vi "Reanimate.vi"(4 "Hook Search Path":path[](array[path]), 6 "Execute Hooks?":cluster{"Pre":bool, "Post":bool}={"Pre"=TRUE, "Post"=TRUE}, 8 "Error In":errorcluster, 10 "Graves":refnum<vi>[](array[refnum]), 11 "VI In":refnum<vi>) -> (0 "Error Out":errorcluster, 2 "Change Made?":bool, 3 "VI Out":refnum<vi>)   [LabVIEW 2018, in "Toolkit.lvlib"]
doc: "Creates zombies at each grave. Enables the Corpse (legacy) frame and disables the Spirit (refactored) frame of each grave. A grave is Diagram Disable Structure with a RIP bookmark tag for its label, a.k.a. tombstone. The Corpse (legacy) frame's subdiagram label is changed from \"Corpse\" to a Zombie bookmark tag with an ISO-8601 timestamp for its \"rebirthday\" and the user that created the zombie, a.k.a. the necromancer, surrounded by parentheses."
uses:
  Toolkit.lvlib
  Typedefs/Bookmark Tags.ctl
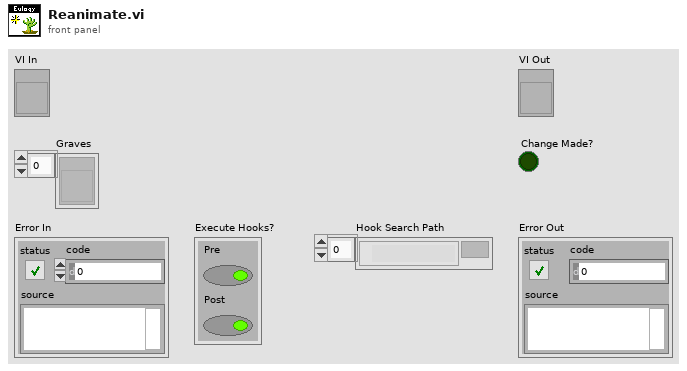
[diagram p1: front panel]
types:
  T1 = typedef "Toolkit.lvlib/Bookmark Tags.ctl" = enum16{"RIP", "Zombie"}
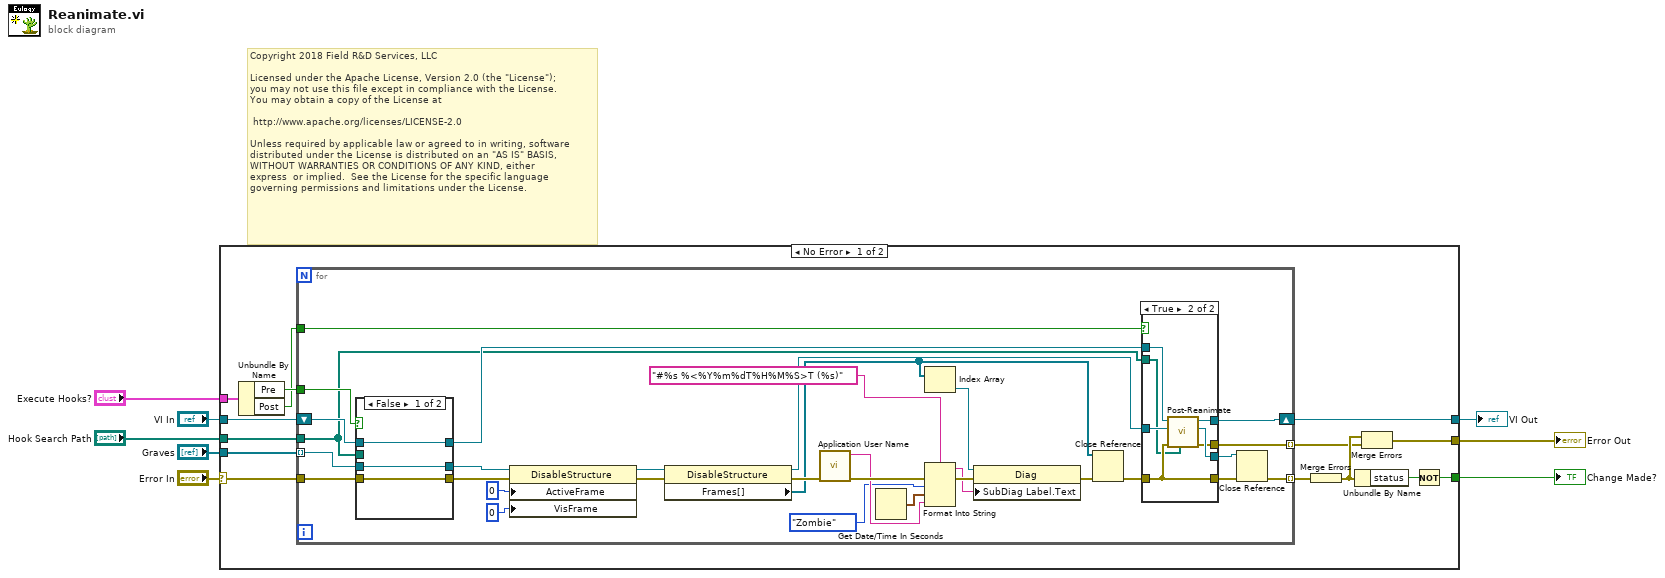
[diagram p0: block diagram]
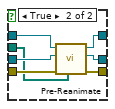
[diagram p3: hidden frame]
diagram:
  # "Copyright 2018 Field R&D Services, LLC\n\nLicensed under the Apache License, Version 2.0 (the \"License\");\nyou may not use this file except in compliance with the License.\nYou may obtain a copy of the License at\n\n\thttp://www.apache.org/licenses/LICENSE-2.0\n\nUnless required by applicable law or agreed to in writing, software\ndistributed under the License is distributed on an \"AS IS\" BASIS,\nWITHOUT WARRANTIES OR CONDITIONS OF ANY KIND, either \nexpress  or implied.  See the License for the specific language \ngoverning permissions and limitations under the License."
  n1 = case shown="No Error" "Error In" {
    selector: "Error In" -> [w21 w75]
    tunnel: [w9 w75] -> w8
    tunnel: "Graves" -> [w22 _]
    tunnel: [w18 _] -> w5
    tunnel: "VI In" -> [w17 w74]
    tunnel: [w16 w74] -> w3
    tunnel: "Execute Hooks?" -> [w15 _]
    tunnel: "Hook Search Path" -> [w13 _]
    frame No Error {
      n2 = Unbundle By Name(w15) -> ("Pre"=w14:bool, "Post"=w12:bool)
      n3 = for {
        tunnel: w22 -> [w27] mode=indexing
        tunnel: w21 -> [w37]
        tunnel: [w39] -> w20 mode=indexing
        shift-right: [w30] -> w16
        shift-left: w17 -> [w36]
        tunnel: w14 -> [w38]
        tunnel: w13 -> [w24]
        tunnel: w12 -> [w32]
        tunnel: [w25] -> w10 mode=indexing
        n4 = case shown="False" w38 {
          tunnel: w37 -> [w65 w68]
          tunnel: w36 -> [w66 w73]
          tunnel: [w66 w72] -> w31
          tunnel: [w65 w71] -> w35
          tunnel: w27 -> [w64 w70]
          tunnel: [w64 w69] -> w26
          tunnel: w24 -> [_ w67]
          frame False {
          }
          frame True {
            n5 = call "Pre-Reanimate.vi"("Search Path"=w67, "Error In"=w68, "Grave In"=w70, "VI In"=w73) -> ("Error Out"=w71:errorcluster, "Grave Out"=w69:refnum<vi>, "VI Out"=w72:refnum<vi>)  [unwired: 5 in]
          }
        }
        n6 = property class="DisableStructure"(reference=w26, error in=w35, "ActiveFrame"=i16 0 ("Active Frame"), "VisFrame"=u32 0 ("Visible Frame")) -> (reference out=w53:refnum<vi>, error out=w52:errorcluster)
        n7 = property class="DisableStructure"(reference=w53, error in=w52) -> (reference out=w29:refnum<vi>, error out=w48:errorcluster, "Frames[]"=w23:refnum<vi>[])
        n8 = call "Application User Name.vi"("Error In"=w48) -> ("Error Out"=w47:errorcluster, "User Name"=w44:string)  [unwired: 9 in]
        n9 = Get Date/Time In Seconds() -> (seconds since 1Jan1904=w45:timestamp)
        n10 = Index Array(array=w23) -> (element=w40:refnum<vi>)  [unwired: 1 in]
        n11 = Format Into String(format string="#%s %<%Y%m%dT%H%M%S>T (%s)" ("time format string (%c)"), error in=w47, Bookmark_Tags."Zombie" ("Bookmark"), w45, w44) -> (resulting string=w46:string, error out=w50:errorcluster)  [unwired: 1 in]
        n12 = property class="Diag"(reference=w40, error in=w50, "SubDiag Label.Text"=w46) -> (error out=w51:errorcluster)  [unwired: 1 out]
        n13 = Close Reference(reference=w23, error in (no error)=w51) -> (error out=w34:errorcluster)
        n14 = case shown="True" w32 {
          tunnel: w34 -> [w56 w59]
          tunnel: [w56 w59] -> w33
          tunnel: w31 -> [w55 w62]
          tunnel: [w55 w63] -> w30
          tunnel: w29 -> [w54 w61]
          tunnel: [w54 w60] -> w28
          tunnel: [_ w58] -> w25
          tunnel: w24 -> [_ w57]
          frame False {
          }
          frame True {
            n15 = call "Post-Reanimate.vi"("Search Path"=w57, "Error In"=w59, "Grave In"=w61, "VI In"=w62) -> ("Error Out"=w58:errorcluster, "Grave Out"=w60:refnum<vi>, "VI Out"=w63:refnum<vi>)  [unwired: 5 in]
          }
        }
        n16 = Close Reference(reference=w28, error in (no error)=w33) -> (error out=w39:errorcluster)
      }
      n17 = Merge Errors(w20) -> (w11:errorcluster)
      n18 = Unbundle By Name(w11) -> ("status"=w19:bool)
      n19 = Merge Errors(w11, w10) -> (w9:errorcluster)
      n20 = Not(x=w19) -> (.not. x?=w18:bool)
    }
    frame Error {
    }
  }
  "Error Out" <- w8
  "Change Made?" <- w5
  "VI Out" <- w3
